vi "Pockels Cal-Automation module.vi"(9 "Timed out":bool, 11 "Pockels control voltage index":i32) -> (0 "error out":errorcluster, 1 "Abort this objective":bool, 2 "Cancelled":bool, 3 "Measured power":dbl, 4 "Timed out or errored out":bool)   [LabVIEW 2020]
uses:
  Globals/gl_Calibration globals.vi
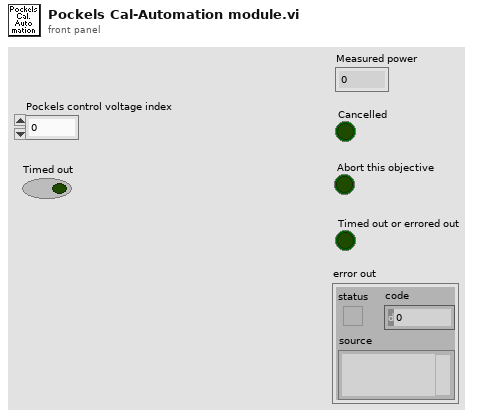
[diagram p1: front panel]
types:
  T1 = typedef "Pockels cal process refs.ctl" = cluster{"This VI":refnum<vi>, "Abort (ind)":refnum<vi>, "Next (ind)":refnum<vi>, "Cancel":refnum<vi>, "Next":refnum<vi>, "Message":refnum<vi>, "Measured Power ctrl":refnum<vi>, "Measured Power ind":refnum<vi>, "Pockels cal progress bar":refnum<vi>, "Abort this objective":refnum<vi>}
  T2 = typedef "Cal mode.ctl" = enum16{"Automatic", "Interactive"}
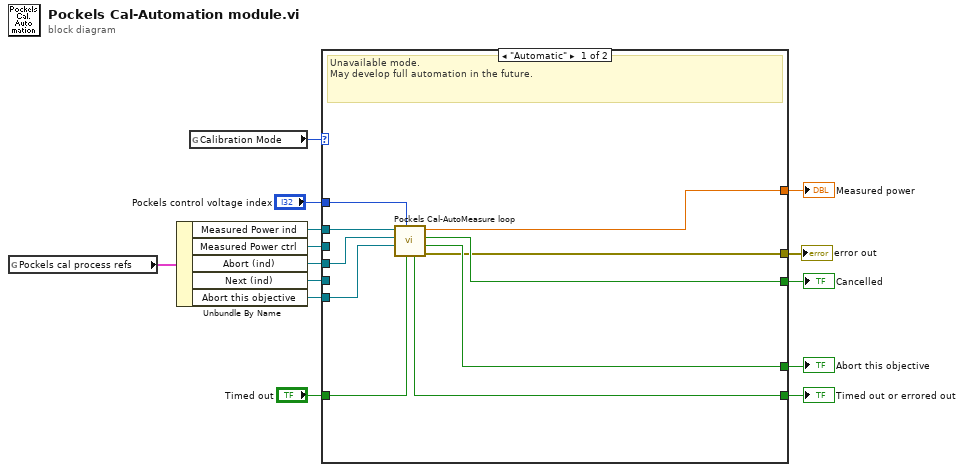
[diagram p0: block diagram]
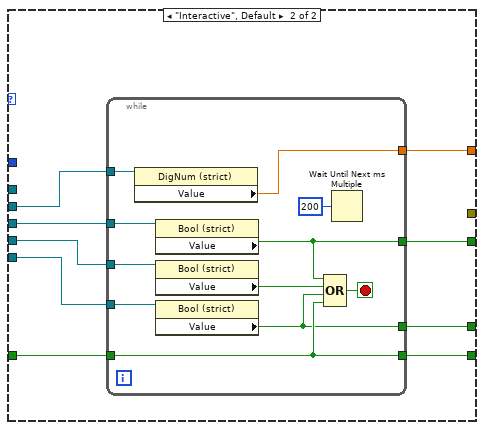
[diagram p2: hidden frame]
diagram:
  n1 = global read "gl_Calibration globals.vi" "Pockels cal process refs"() -> (w9:T1)
  n2 = Unbundle By Name(w9) -> ("Measured Power ind"=w3:refnum<vi>, "Measured Power ctrl"=w6:refnum<vi>, "Abort (ind)"=w13:refnum<vi>, "Next (ind)"=w14:refnum<vi>, "Abort this objective"=w5:refnum<vi>)
  n3 = global read "gl_Calibration globals.vi" "Calibration Mode"() -> (w7:T2)
  n4 = case shown="\"Automatic\"" w7 {
    tunnel: w14 -> [_ w33]
    tunnel: w13 -> [w23 w32]
    tunnel: [w18 w31] -> w12
    tunnel: "Timed out" -> [w17 w30]
    tunnel: [w22 w29] -> w10
    tunnel: [w19 w28] -> w8
    tunnel: w6 -> [_ w27]
    tunnel: w5 -> [w21 w26]
    tunnel: [w20 w25] -> w4
    tunnel: w3 -> [w24 _]
    tunnel: [w16 _] -> w2
    tunnel: "Pockels control voltage index" -> [w15 _]
    frame "Automatic" {
      # "Unavailable mode.\nMay develop full automation in the future."
      n5 = call "Pockels Cal-AutoMeasure loop.vi"("Timed out (in)"=w17, "Pockels control voltage index"=w15, "Abort this objective"=w21, "Abort"=w23, "Measured power ind"=w24) -> ("error out"=w16:errorcluster, "Abort this objective"=w20:bool, "Aborted"=w22:bool, "Measured power (mW)"=w19:dbl, "Timed out"=w18:bool)  [unwired: 2 in]
    }
    frame "Interactive", Default {
      n6 = while {
        tunnel: w33 -> [w44]
        tunnel: w32 -> [w43]
        tunnel: [w36] -> w31
        tunnel: w30 -> [w36]
        tunnel: [w42] -> w29
        tunnel: [w37] -> w28
        tunnel: w27 -> [w38]
        tunnel: w26 -> [w35]
        tunnel: [w34] -> w25
        stop <- w40 stop-if-true
        n7 = property class="DigNum (strict)"(reference=w38) -> ("Value"=w37:dbl)  [unwired: 1 in, 2 out]
        n8 = property class="Bool (strict)"(reference=w43) -> ("Value"=w42:bool)  [unwired: 1 in, 2 out]
        n9 = property class="Bool (strict)"(reference=w44) -> ("Value"=w41:bool)  [unwired: 1 in, 2 out]
        n10 = property class="Bool (strict)"(reference=w35) -> ("Value"=w34:bool)  [unwired: 1 in, 2 out]
        n11 = Compound Arithmetic op=OR(w42, w41, w34, w36) -> (w40:bool)
        n12 = Wait Until Next ms Multiple(millisecond multiple=u32 200) -> ()  [unwired: 1 out]
      }
    }
  }
  "Timed out or errored out" <- w12
  "Cancelled" <- w10
  "Measured power" <- w8
  "Abort this objective" <- w4
  "error out" <- w2
